vi "Sequence.Tools.FinalStatus.vi"(1 "Status array":T1[](array[typedef])) -> (0 "Final Status":T1)   [LabVIEW 2016]
uses:
  Sequence.Step.Status.ctl
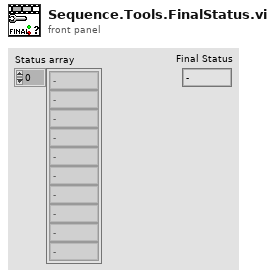
[diagram p1: front panel]
types:
  T1 = typedef "Sequence.Step.Status.ctl" = enum16{"-", "Pending", "Running", "Skipped", "Passed", "Failed", "Done", "Error", "Aborted", "Stopped"}
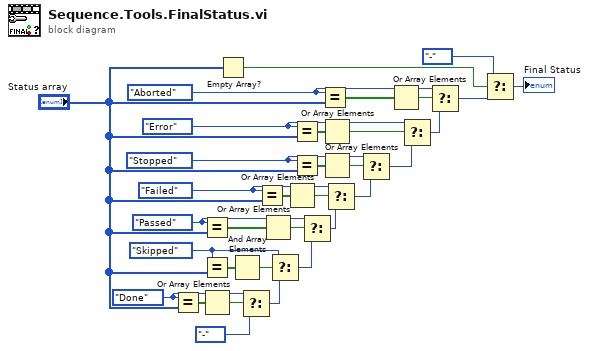
[diagram p0: block diagram]
diagram:
  w8 = Sequence.Step.Status."Done" ("y")
  w13 = Sequence.Step.Status."Stopped" ("y")
  w17 = Sequence.Step.Status."Skipped" ("y")
  w33 = Sequence.Step.Status."Passed" ("y")
  w32 = Sequence.Step.Status."Failed" ("y")
  w31 = Sequence.Step.Status."Error" ("y")
  w30 = Sequence.Step.Status."Aborted" ("y")
  n1 = Equal?(x=w8, y="Status array") -> (x = y?=w9:bool[])
  n2 = Equal?(x=w33, y="Status array") -> (x = y?=w28:bool[])
  n3 = Equal?(x=w17, y="Status array") -> (x = y?=w19:bool[])
  n4 = Or Array Elements(Boolean array=w9) -> (logical OR=w10:bool)
  n5 = Empty Array?(array="Status array") -> (empty?=w3:bool)
  n6 = And Array Elements(Boolean array=w19) -> (logical AND=w18:bool)
  n7 = Select(t=w8, s=w10, f=Sequence.Step.Status."-" ("y")) -> (s? t:f=w7:T1)
  n8 = Equal?(x=w32, y="Status array") -> (x = y?=w25:bool[])
  n9 = Or Array Elements(Boolean array=w28) -> (logical OR=w27:bool)
  n10 = Select(t=w17, s=w18, f=w7) -> (s? t:f=w16:T1)
  n11 = Or Array Elements(Boolean array=w25) -> (logical OR=w26:bool)
  n12 = Equal?(x=w31, y="Status array") -> (x = y?=w23:bool[])
  n13 = Equal?(x=w13, y="Status array") -> (x = y?=w15:bool[])
  n14 = Select(t=w33, s=w27, f=w16) -> (s? t:f=w29:T1)
  n15 = Equal?(x=w30, y="Status array") -> (x = y?=w20:bool[])
  n16 = Or Array Elements(Boolean array=w23) -> (logical OR=w22:bool)
  n17 = Or Array Elements(Boolean array=w15) -> (logical OR=w14:bool)
  n18 = Select(t=w32, s=w26, f=w29) -> (s? t:f=w12:T1)
  n19 = Select(t=w13, s=w14, f=w12) -> (s? t:f=w11:T1)
  n20 = Or Array Elements(Boolean array=w20) -> (logical OR=w21:bool)
  n21 = Select(t=w31, s=w22, f=w11) -> (s? t:f=w24:T1)
  n22 = Select(t=w30, s=w21, f=w24) -> (s? t:f=w4:T1)
  n23 = Select(t=Sequence.Step.Status."-" ("y"), s=w3, f=w4) -> (s? t:f=→"Final Status":T1)
